vi "Show Labels.vi"(8 "error in (no error)":errorcluster, 11 "VI Reference In":refnum<vi>) -> (0 "error out":errorcluster, 3 "VI Reference Out":refnum<vi>)   [LabVIEW 2021]
panel:
  # "This VI takes a reference to the scripted VI and turns on the \n\"Label.Visible\" property on all constants in the scripted block \ndiagram"
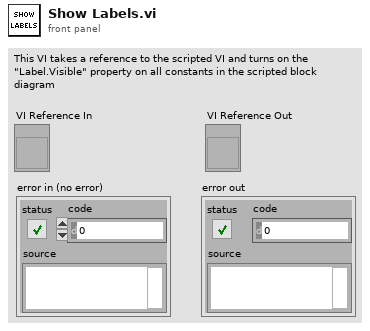
[diagram p1: front panel]
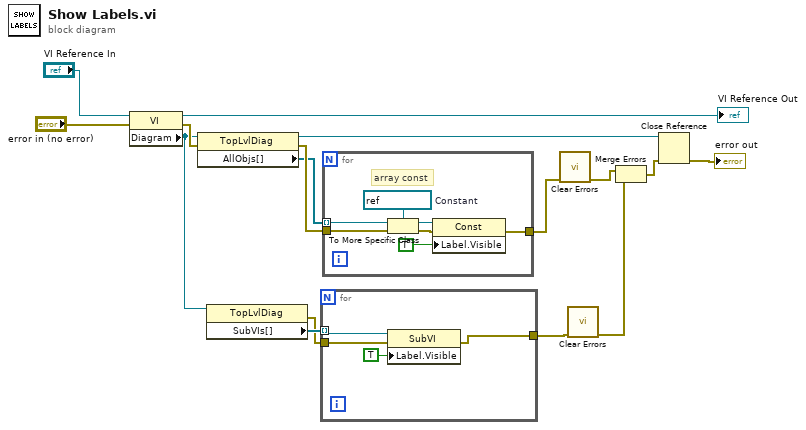
[diagram p0: block diagram]
diagram:
  n1 = property class="VI"(reference="VI Reference In", error in="error in (no error)") -> (reference out=→"VI Reference Out":refnum<vi>, error out=w15:errorcluster, "Diagram"=w7:refnum<vi>)
  n2 = property class="TopLvlDiag"(reference=w7, error in=w15) -> (reference out=w13:refnum<vi>, error out=w12:errorcluster, "AllObjs[]"=w10:refnum<vi>[])
  n3 = property class="TopLvlDiag"(reference=w7) -> (error out=w5:errorcluster, "SubVIs[]"=w6:refnum<vi>[])  [unwired: 1 in, 1 out]
  n4 = for {
    tunnel: w6 -> [w20] mode=indexing
    tunnel: w5 -> [w19]
    tunnel: [w18] -> w4
    n5 = property class="SubVI"(reference=w20, error in=w19, "Label.Visible"=TRUE) -> (error out=w18:errorcluster)  [unwired: 1 out]
  }
  n6 = for {
    tunnel: w10 -> [w25] mode=indexing
    tunnel: [w22] -> w11
    tunnel: w12 -> [w21]
    w27 = refnum<vi> refnum  # Constant
    # "array const"
    n7 = To More Specific Class(target class=w27, reference=w25, error in=w21) -> (specific class reference=w26:refnum<vi>, error out=w23:errorcluster)
    n8 = property class="Const"(reference=w26, error in=w23, "Label.Visible"=TRUE ("Size To Text?")) -> (error out=w22:errorcluster)  [unwired: 1 out]
  }
  n9 = call <vilib>:"Clear Errors.vi"("error in (no error)"=w11) -> ("error out"=w2:errorcluster)  [unwired: 5 in, 1 out]
  n10 = call <vilib>:"Clear Errors.vi"("error in (no error)"=w4) -> ("error out"=w1:errorcluster)  [unwired: 5 in, 1 out]
  n11 = Merge Errors(w2, w1) -> (w3:errorcluster)
  n12 = Close Reference(reference=w13, error in (no error)=w3) -> (error out=→"error out":errorcluster)
